vi "例题5.3.vi"() -> ()   [LabVIEW 2017]
panel:
  out "数组":dbl[](array[numeric])
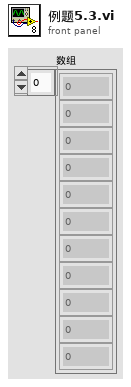
[diagram p1: front panel]
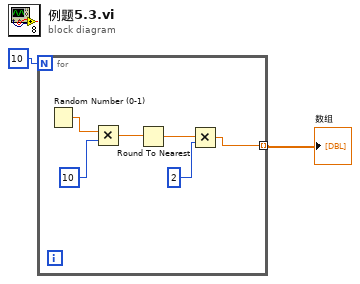
[diagram p0: block diagram]
diagram:
  n1 = for {
    N: 10 -> [_]
    tunnel: [w5] -> w1 mode=indexing
    n2 = Random Number (0-1)() -> (number: 0 to 1=w4:dbl)
    n3 = Multiply(x=w4, y=10) -> (x*y=w8:dbl)
    n4 = Round To Nearest(number=w8) -> (nearest integer value=w7:dbl)
    n5 = Multiply(x=w7, y=2) -> (x*y=w5:dbl)
  }
  "数组" <- w1
